vi "sub_pf_motion-model.vi"(6 "Real Matrix":T1, 9 "rf_id":cluster{"x":dbl, "y":dbl}[](array[cluster]), 10 "x_dr":T1, 11 "x_true":T1) -> (2 "B":T1, 3 "ぜ":T1 caption="A + B")   [LabVIEW 2019]
uses:
  <vilib>/Analysis/Matrix/Datatypes/RealMatrix.ctl
  Ctrl/cmd_common.ctl
  <vilib>/Analysis/Matrix/Numeric/Multiply/Multiply - RM,RM.vi
  <vilib>/Analysis/Matrix/Numeric/Add/Add - RM,RM.vi
  <vilib>/Analysis/Matrix/NI_Matrix.lvlib
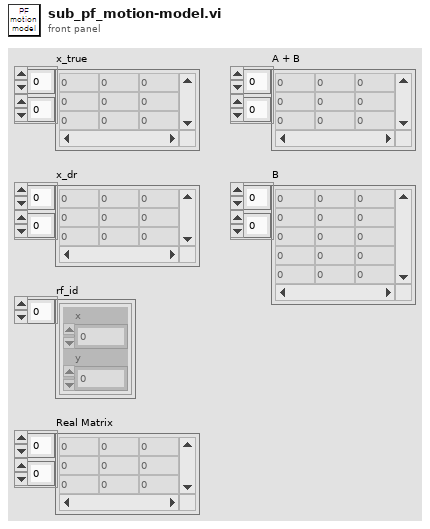
[diagram p1: front panel]
types:
  T1 = typedef "NI_Matrix.lvlib/RealMatrix.ctl" = dbl[][]
  T2 = typedef "cmd_common.ctl" = enum16{"read", "write"}
  T3 = cluster{"DT":dbl, "SIM_TIME":dbl, "MAX_RANGE":dbl, "NP":u32, "NTh":dbl, "Q_sim":T1, "R_sim":T1}
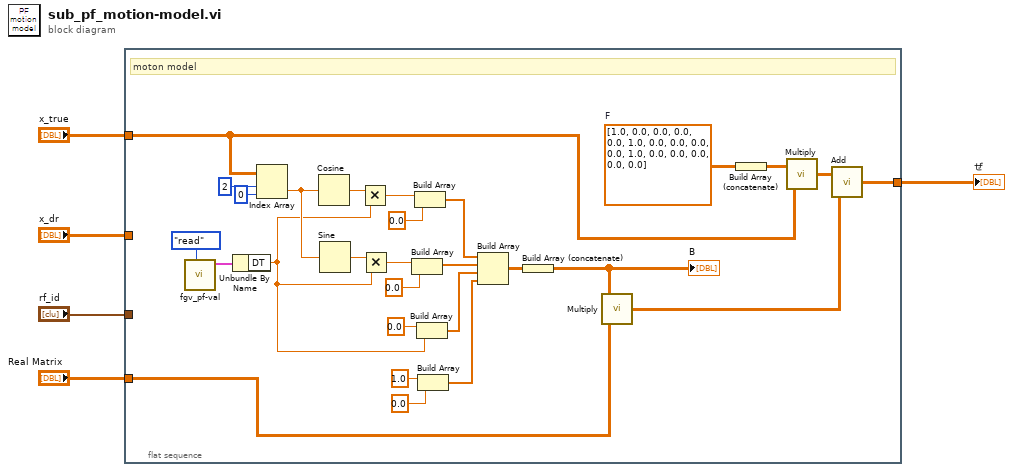
[diagram p0: block diagram]
diagram:
  n1 = flat-sequence {
    tunnel: "x_true" -> [w12]
    tunnel: "Real Matrix" -> [w10]
    tunnel: "x_dr" -> [_]
    tunnel: "rf_id" -> [_]
    tunnel: [w6] -> w5
    frame #0 {
      w14 = dbl[][] [[1.0, 0.0, 0.0, 0.0], [0.0, 1.0, 0.0, 0.0], [0.0, 0.0, 1.0, 0.0], [0.0, 0.0, 0.0, 0.0]]  # F
      # "moton model"
      n2 = call "fgv_pf-val.vi"("cmd"=cmd_common."read") -> ("pf-val out"=w8:T3)  [unwired: 10 in]
      n3 = Unbundle By Name(w8) -> ("DT"=w7:dbl)
      n4 = Index Array(array=w12, index (row)=2 ("인덱스 (행)"), index (col)=0 ("인덱스 (열)")) -> (element=w29:dbl)
      n5 = Cosine(x=w29) -> (cos(x)=w31:dbl)
      n6 = Sine(x=w29) -> (sin(x)=w30:dbl)
      n7 = Multiply(x=w31, y=w7) -> (x*y=w28:dbl)
      n8 = Multiply(x=w30, y=w7) -> (x*y=w25:dbl)
      n9 = Build Array(w25, 0.0 ("원소")) -> (w19:dbl[])
      n10 = Build Array(w28, 0.0 ("원소")) -> (w18:dbl[])
      n11 = Build Array(0.0 ("원소"), w7) -> (w20:dbl[])
      n12 = Build Array(1.0 ("원소"), 0.0 ("원소")) -> (w21:dbl[])
      n13 = Build Array(w18, w19, w20, w21) -> (w17:dbl[][])
      n14 = Build Array (concatenate)(w17) -> (w16:T1)
      "B" <- w16
      n15 = call-poly <vilib>:"Multiply.vi"("Real Matrix B"=w10, "Real Matrix A"=w16) -> ("A * B"=w15:T1)
      n16 = Build Array (concatenate)(w14) -> (w13:T1)
      n17 = call-poly <vilib>:"Multiply.vi"("Real Matrix B"=w12, "Real Matrix A"=w13) -> ("A * B"=w11:T1)
      n18 = call-poly <vilib>:"Add.vi"("Real Matrix B"=w15, "Real Matrix A"=w11) -> ("A + B"=w6:T1)
    }
  }
  "ぜ" <- w5
